vi "DoCalibration.vi"(8 "Offsets":dbl[](array[numeric]), 9 "Slopes":dbl[](array[numeric]), 10 "Channel Tags":string[](array[string]), 11 "Data":T1 caption="All Data Cluster") -> (3 "DataOut":T1 caption="All Data Cluster")   [LabVIEW 2018, in "Controller (Host).lvlib"]
uses:
  Controller (Host).lvlib
  Top Level/Shared Controls/All Data Cluster.ctl
  Top Level/Shared Controls/Acq Data.ctl
  <vilib>/Utility/error.llb/Error Cluster From Error Code.vi
  <vilib>/ErrorRing/Error Ring.xnode
panel:
  in  "ErrorIn":errorcluster
  out "ErrorOut":errorcluster
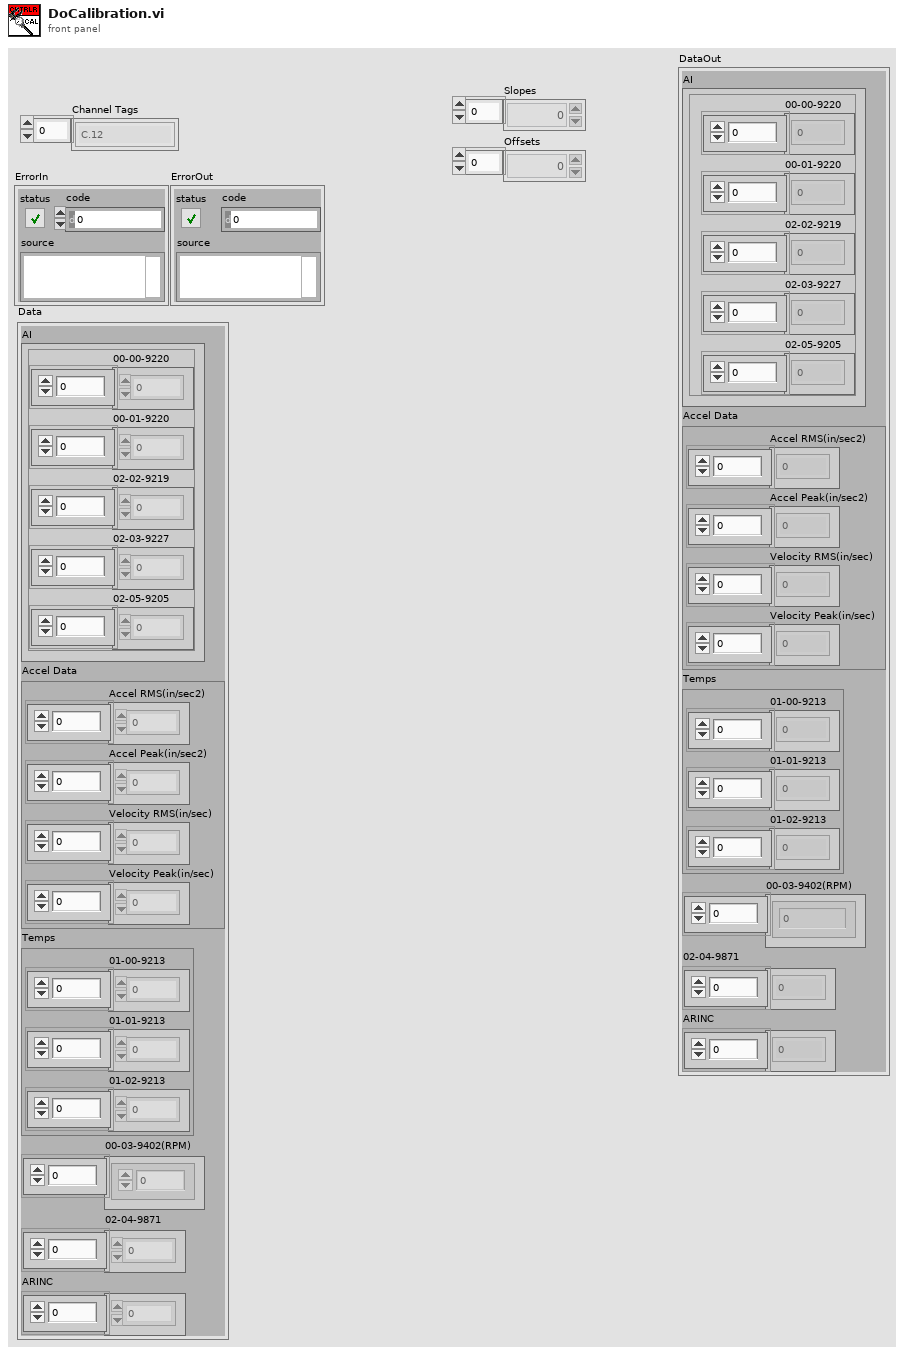
[diagram p1: front panel]
types:
  T1 = typedef "All Data Cluster.ctl" = cluster{"AI":T2, "Accel Data":cluster{"Accel RMS(in/sec2)":dbl[], "Accel Peak(in/sec2)":dbl[], "Velocity RMS(in/sec)":dbl[], "Velocity Peak(in/sec)":dbl[]}, "Temps":cluster{"01-00-9213":dbl[], "01-01-9213":dbl[], "01-02-9213":dbl[]}, "00-03-9402(RPM)":dbl[], "02-04-9871":dbl[], "ARINC":sgl[]}
  T2 = typedef "Acq Data.ctl" = cluster{"00-00-9220":dbl[], "00-01-9220":dbl[], "02-02-9219":dbl[], "02-03-9227":dbl[], "02-05-9205":dbl[]}
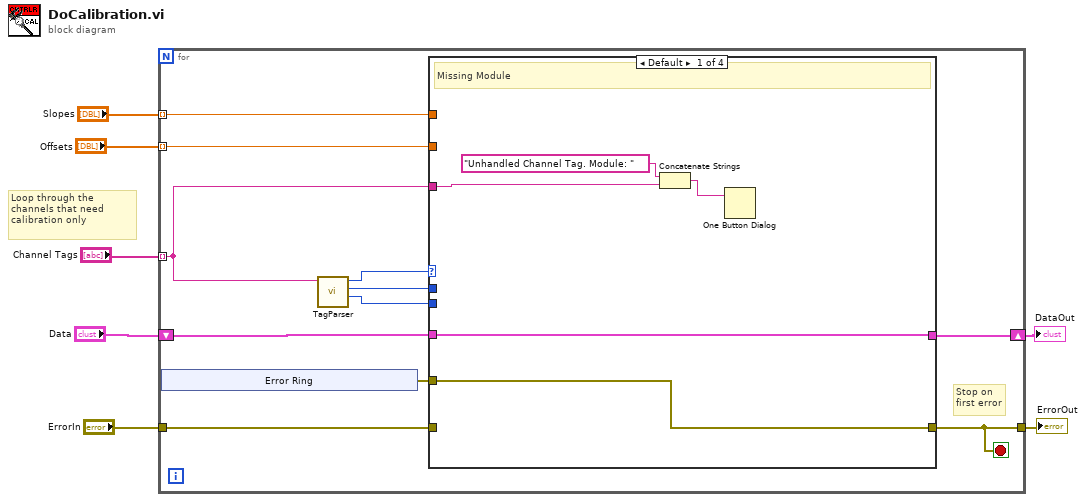
[diagram p0: block diagram]
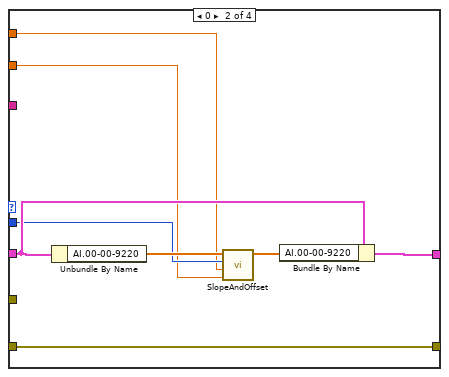
[diagram p3: hidden frame]
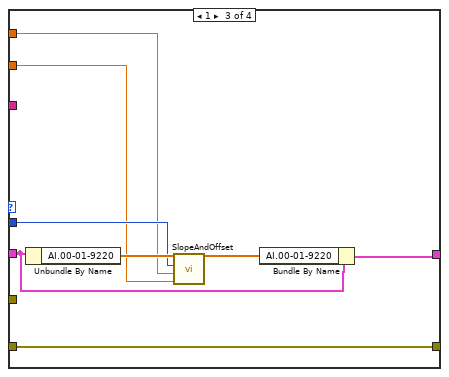
[diagram p4: hidden frame]
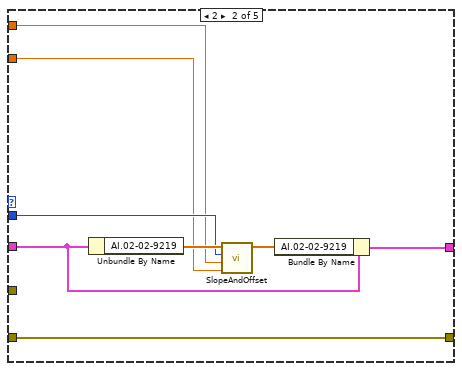
[diagram p9: hidden frame]
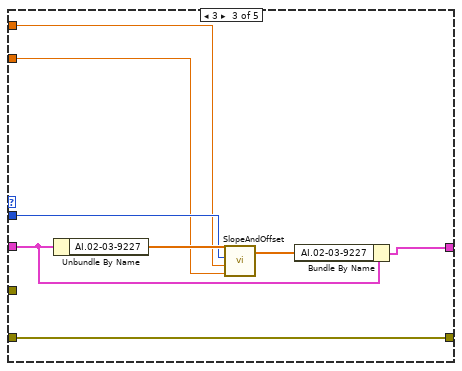
[diagram p10: hidden frame]
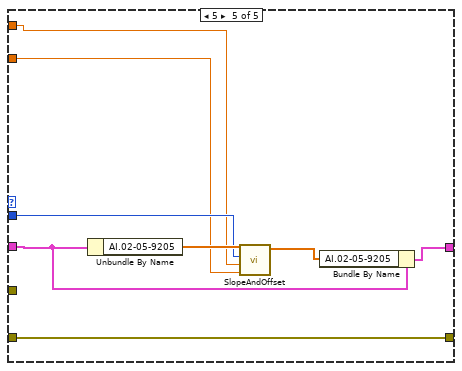
[diagram p11: hidden frame]
diagram:
  # "Loop through the channels that need calibration only"
  n1 = for {
    tunnel: "Channel Tags" -> [w8] mode=indexing
    tunnel: "ErrorIn" -> [w18]
    tunnel: [w16] -> w7
    tunnel: "Slopes" -> [w11] mode=indexing
    tunnel: "Offsets" -> [w10] mode=indexing
    shift-right: [w9] -> w1
    shift-left: "Data" -> [w15]
    stop <- w16 stop-if-true
    # "Stop on\nfirst error"
    n2 = xnode "Error Ring"() -> ("error out"=w17:errorcluster)
    n3 = call "TagParser.vi"("Channel Tag"=w8) -> ("Channel"=w12:i32, "Module"=w13:i32, "Chassis"=w14:i32)  [unwired: 8 in]
    n4 = case shown="Default" w14 {
      tunnel: w13 -> [_ w33 _ w63]
      tunnel: w15 -> [w19 w32 w55 w62]
      tunnel: w12 -> [_ w31 _ w64]
      tunnel: w18 -> [_ w30 w54 w61]
      tunnel: w17 -> [w21 w29 _ w59]
      tunnel: [w21 w28 w54 w60] -> w16
      tunnel: w11 -> [_ w26 _ w58]
      tunnel: w10 -> [_ w27 _ w57]
      tunnel: [w19 w25 w55 w56] -> w9
      tunnel: w8 -> [w20 w24 _ _]
      frame Default {
        # "Missing Module"
        n5 = Concatenate Strings("Unhandled Channel Tag. Module: " ("message"), w20) -> (w22:string)
        n6 = One Button Dialog(message=w22) -> ()  [unwired: 1 in, 1 out]
      }
      frame 0 {
        # "Chassis 0"
        n7 = case shown="Default" w33 {
          tunnel: w32 -> [w34 w42 w46 w52]
          tunnel: w31 -> [_ w38 w49 _]
          tunnel: w30 -> [_ w43 w51 w53]
          tunnel: w29 -> [w35 _ _ _]
          tunnel: [w35 w43 w51 w53] -> w28
          tunnel: w27 -> [_ w36 w47 _]
          tunnel: w26 -> [_ w37 w48 _]
          tunnel: [w34 w40 w44 w52] -> w25
          tunnel: w24 -> [_ _ _ _]
          frame Default {
          }
          frame 0 {
            n8 = Unbundle By Name(w42) -> ("AI.00-00-9220"=w39:dbl[])
            n9 = call "SlopeAndOffset.vi"("Offset"=w36, "Slope"=w37, "Index"=w38, "Data in"=w39) -> ("Data out"=w41:dbl[])  [unwired: 7 in]
            n10 = Bundle By Name(cluster=w42, "AI.00-00-9220"=w41) -> (w40:T1)
          }
          frame 1 {
            n11 = Unbundle By Name(w46) -> ("AI.00-01-9220"=w50:dbl[])
            n12 = call "SlopeAndOffset.vi"("Offset"=w47, "Slope"=w48, "Index"=w49, "Data in"=w50) -> ("Data out"=w45:dbl[])  [unwired: 7 in]
            n13 = Bundle By Name(cluster=w46, "AI.00-01-9220"=w45) -> (w44:T1)
          }
          frame 3 {
            # "No Calibration Required"
          }
        }
      }
      frame 1 {
        # "No Cal Required. All Temps"
        # "Chassis 1"
      }
      frame 2 {
        # "CHASSIS 2"
        n14 = case shown="4" w63 {
          tunnel: w62 -> [w65 w69 w77 w83 w87]
          tunnel: w64 -> [_ w72 w80 _ w90]
          tunnel: w61 -> [_ w74 w82 w84 w92]
          tunnel: [w66 w74 w82 w84 w92] -> w60
          tunnel: w59 -> [w66 _ _ _ _]
          tunnel: w58 -> [_ w71 w79 _ w89]
          tunnel: w57 -> [_ w70 w78 _ w88]
          tunnel: [w65 w67 w75 w83 w85] -> w56
          frame Default {
          }
          frame 2 {
            n15 = Unbundle By Name(w69) -> ("AI.02-02-9219"=w73:dbl[])
            n16 = call "SlopeAndOffset.vi"("Offset"=w70, "Slope"=w71, "Index"=w72, "Data in"=w73) -> ("Data out"=w68:dbl[])  [unwired: 7 in]
            n17 = Bundle By Name(cluster=w69, "AI.02-02-9219"=w68) -> (w67:T1)
          }
          frame 3 {
            n18 = Unbundle By Name(w77) -> ("AI.02-03-9227"=w81:dbl[])
            n19 = call "SlopeAndOffset.vi"("Offset"=w78, "Slope"=w79, "Index"=w80, "Data in"=w81) -> ("Data out"=w76:dbl[])  [unwired: 7 in]
            n20 = Bundle By Name(cluster=w77, "AI.02-03-9227"=w76) -> (w75:T1)
          }
          frame 4 {
            # "Modbus. No Cal Required."
          }
          frame 5 {
            n21 = Unbundle By Name(w87) -> ("AI.02-05-9205"=w91:dbl[])
            n22 = call "SlopeAndOffset.vi"("Offset"=w88, "Slope"=w89, "Index"=w90, "Data in"=w91) -> ("Data out"=w86:dbl[])  [unwired: 7 in]
            n23 = Bundle By Name(cluster=w87, "AI.02-05-9205"=w86) -> (w85:T1)
          }
        }
      }
    }
  }
  "ErrorOut" <- w7
  "DataOut" <- w1
